vi "MTMount_getEvent_softwareVersions.vi"(8 "error in (no error)":errorcluster, 11 "logevent_softwareVersions_Ctl":T1={"salVersion"="", "xmlVersion"="", "openSpliceVersion"="                ", "cscVersion"="", "subsystemVersions"="", "priority"=0}) -> (0 "error out":errorcluster, 2 "function return":i32, 3 "logevent_softwareVersions_Ctl out":T1={"salVersion"="", "xmlVersion"="", "openSpliceVersion"="                ", "cscVersion"="", "subsystemVersions"="", "priority"=0})   [LabVIEW 2018, in "SALLV_MTMount.lvlib"]
doc: "int MTMount_shm_getEvent_softwareVersionsLV(MTMount_logevent_softwareVersionsLV *logevent_softwareVersions_Ctl );"
uses:
  SALLV_MTMount.lvlib
  DataTypes/logevent_softwareVersions.ctl
  SALLV_MTMount.so
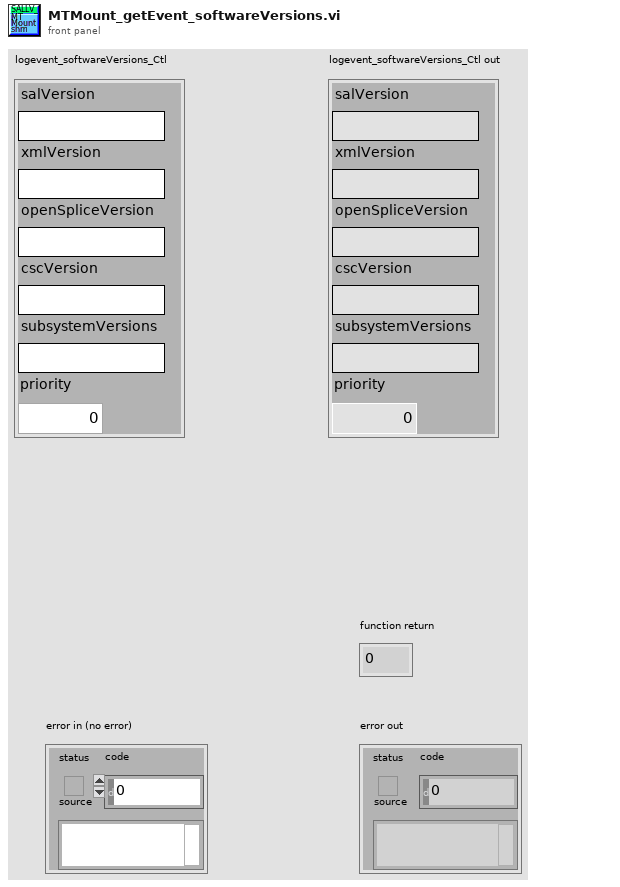
[diagram p1: front panel]
types:
  T1 = typedef "SALLV_MTMount.lvlib/logevent_softwareVersions.ctl" = cluster{"salVersion":string, "xmlVersion":string, "openSpliceVersion":string, "cscVersion":string, "subsystemVersions":string, "priority":i32}
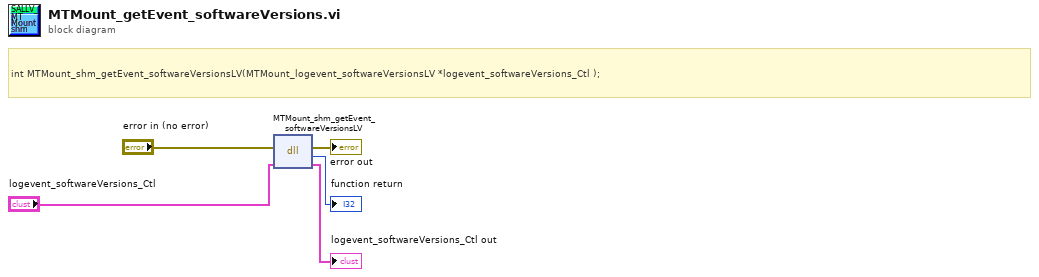
[diagram p0: block diagram]
diagram:
  # "int MTMount_shm_getEvent_softwareVersionsLV(MTMount_logevent_softwareVersionsLV *logevent_softwareVersions_Ctl );"
  n1 = dll-call lib="home/ttsai/Document/salApiMTMount/SALLV_MTMount/SALLV_MTMount.*" fn="MTMount_shm_getEvent_softwareVersionsLV"(error in="error in (no error)", "logevent_softwareVersions_Ctl"="logevent_softwareVersions_Ctl") -> (error out=→"error out":errorcluster, →"function return":i32, "logevent_softwareVersions_Ctl"=→"logevent_softwareVersions_Ctl out":T1)  [unwired: 2 in, 1 out]
